vi "Test Parse XML Heap.vi"() -> ()   [LabVIEW 2026, in "VILab.lvlib"]
uses:
  VILab.lvlib
  SubVIs/Decompose VI (Refnum).vi
  Classes/Data Item/Data Item.lvclass
panel:
  out "Table Control":string[][](table)
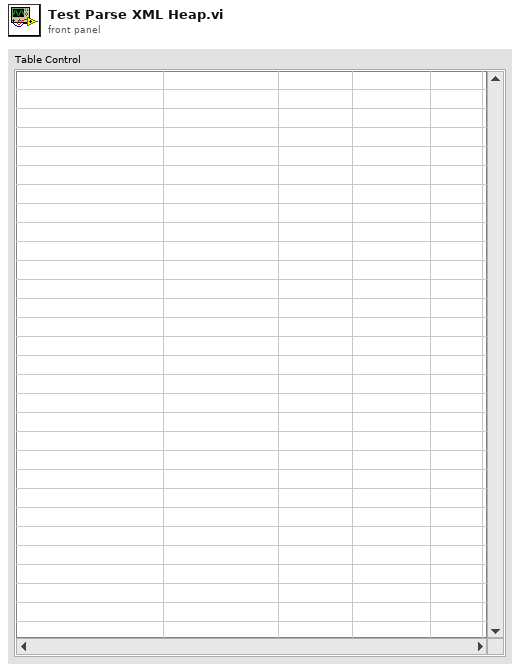
[diagram p1: front panel]
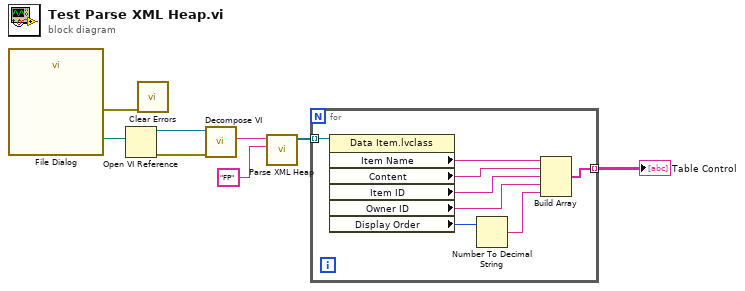
[diagram p0: block diagram]
diagram:
  n1 = call "File Dialog"() -> ("selected path"=w6:path, "error out"=w5:errorcluster)  [unwired: 12 in, 2 out]
  n2 = Open VI Reference(vi path=w6) -> (vi reference=w8:refnum<vi>, error out=w7:errorcluster)  [unwired: 5 in]
  n3 = call <vilib>:"Clear Errors.vi"("error in (no error)"=w5) -> ()  [unwired: 5 in, 2 out]
  n4 = call-poly "Decompose VI.vi"("error in (no error)"=w7, "VI Ref"=w8) -> ("Front Panel XML"=w4:string)  [unwired: 5 in, 4 out]
  n5 = call "Parse XML Heap.vi"("Root Parent"="FP", "XML"=w4) -> ("Items"=w3:refnum<class "Data Item.lvclass">[])  [unwired: 8 in, 1 out]
  n6 = for {
    tunnel: w3 -> [w16] mode=indexing
    tunnel: [w12] -> w2 mode=indexing
    n7 = property class="Data Item.lvclass"(reference=w16) -> ("Item Name"=w15:string, "Content"=w14:string, "Item ID"=w13:string, "Owner ID"=w11:string, "Display Order"=w10:i32)  [unwired: 1 in, 2 out]
    n8 = Number To Decimal String(number=w10) -> (decimal integer string=w9:string)  [unwired: 1 in]
    n9 = Build Array(w15, w14, w13, w11, w9) -> (w12:string[])
  }
  "Table Control" <- w2
